vi "Finalize.vi"(8 "error in":errorcluster, 11 "Rx execution unit in":refnum<class "Rx Execution Unit.lvclass">) -> (0 "error out":errorcluster, 3 "Rx execution unit out":refnum<class "Rx Execution Unit.lvclass">)   [LabVIEW 2020, in "AIM ARINC 429 Engine.lvlib" / "Implementation.lvlib" / "Rx Execution Unit.lvclass"]
uses:
  Rx Execution Unit.lvclass
  C:/Git/niveristand-aim-arinc429-custom-device/Source/Custom Device Support/Engine/Implementation/Execution Unit/Execution Unit.lvclass
  Rx Execution Unit.lvclass/Rx Execution Unit.ctl
  Execution Unit/Execution Unit.lvclass/Execution Unit.ctl
  <instrlib>/AIM GmbH/ARINC-429/subvi/Error Converter (ErrCode or Status).vi
  <instrlib>/AIM GmbH/ARINC-429/subvi/Get Library Path.vi
  <instrlib>/AIM GmbH/ARINC-429/VIs/Library/Api429Lib Error Desc Get.vi
  <instrlib>/AIM GmbH/ARINC-429/subvi/Get Error Number Offset.vi
  <vilib>/Utility/error.llb/Error Cluster From Error Code.vi
  <instrlib>/AIM GmbH/ARINC-429/AIM429LV.lvlib
  Execution Unit/Execution Unit.lvclass
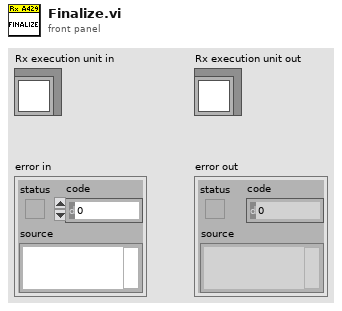
[diagram p1: front panel]
types:
  T1 = typedef "RT Hardware Channel Settings.ctl" = cluster{"channel #":u16, "channel handle":u64, "labels settings for RT":T2[]}
  T2 = typedef "RT Label Settings.ctl" = cluster{"Name":string, "xmlName":string, "label":T3, "transfer period":u32, "SDI_Enabled":bool, "SDI":u8, "parameter driver data":T4, "transfer type":T8, "has timestamp?":bool, "Label Disable/Trigger Channel Reference":T7, "Message Handle":u64, "Initialized?":bool, "Word Initial Raw Value":u32, "Label Timestamp Channel Data Reference":T9, "disabled":bool}
  T3 = typedef "Label.ctl" = u8
  T4 = typedef "RT Parameters.ctl" = cluster{"parameter definitions":T5[], "Tx parameter refs":T7[]}
  T5 = typedef "Parameter Definition.ctl" = cluster{"start index":i32, "size":i32, "encoding":T6, "signed":bool, "scale multiplier":dbl, "scale offset":dbl}
  T6 = typedef "Encoding and Decoding.lvlib/Encoding.ctl" = enum16{"BNR", "BCD", "Discrete"}
  T7 = typedef "Custom Device API.lvlib/Custom Device Item Ref.ctl" = u64
  T8 = typedef "Transfer Type.ctl" = enum16{"Scheduled", "Acyclic", "Block", "Strobe"}
  T9 = typedef "Custom Device API.lvlib/Data Reference.ctl" = i32
  T10 = typedef "AIM ARINC 429 Engine.lvlib/Custom Device.lvlib/Hardware Handles.ctl" = cluster{"module":u8}
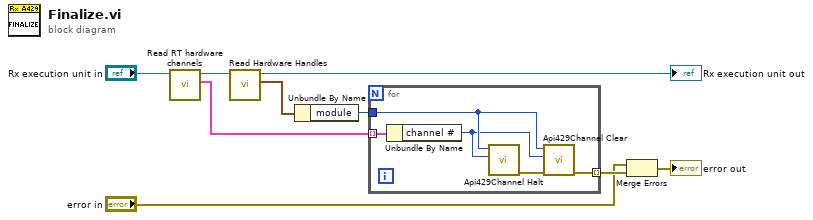
[diagram p0: block diagram]
diagram:
  n1 = call "Read RT hardware channels.vi"("Rx execution unit in"="Rx execution unit in") -> ("RT hardware channels"=w4:T1[], "Rx execution unit out"=w8:refnum<class "Rx Execution Unit.lvclass">)  [unwired: 8 in, 1 out]
  n2 = call "Read Hardware Handles.vi"("AIM ARINC-429 execution unit in"=w8) -> ("hardware handles"=w6:T10, "AIM ARINC-429 execution unit out"=→"Rx execution unit out":refnum<class "Rx Execution Unit.lvclass">)  [unwired: 8 in, 1 out]
  n3 = Unbundle By Name(w6) -> ("module"=w5:u8)
  n4 = for {
    tunnel: w5 -> [w13]
    tunnel: w4 -> [w12] mode=indexing
    tunnel: [w10] -> w3 mode=indexing
    n5 = Unbundle By Name(w12) -> ("channel #"=w11:u16)
    n6 = call <instrlib>:"Api429Channel Halt.vi"("channel_id"=w11, "board_handle"=w13) -> ("error out"=w14:errorcluster)  [unwired: 9 in]
    n7 = call <instrlib>:"Api429Channel Clear.vi"("error in (no error)"=w14, "channel_id"=w11, "board_handle"=w13) -> ("error out"=w10:errorcluster)  [unwired: 8 in]
  }
  n8 = Merge Errors("error in", w3) -> (→"error out":errorcluster)
